vi "LINXx - Analog IO.vi"() -> ()   [LabVIEW 2019]
uses:
  <vilib>/MakerHub/LINX/Public/Peripherals/Analog/Analog Read 1 Chan.vi
  <vilib>/MakerHub/LINX/Public/Peripherals/Analog/Analog Read N Chans.vi
  <vilib>/MakerHub/LINX/Private/Local IO/LinxAnalogRead.vi
  <vilib>/MakerHub/LINX/Public/Utilities/Check Channel.vi
  <vilib>/MakerHub/LINX/Public/Utilities/Open Serial.vi
  <vilib>/MakerHub/LINX/Public/Peripherals/Analog/Analog Write 1 Chan.vi
  <vilib>/MakerHub/LINX/Private/Utilties/Generate Error.vi
  <vilib>/MakerHub/LINX/LMH-LINX.lvlib
  vi.lib/LINXx/LINXx.lvlib
panel:
  in  "AI Channel":u8=15
  in  "AO Channel":u8=14
  in  "iterations per cycle":i32=400
  out "Loop Rate (Hz)":u32
  out "Waveform Chart":cluster{dbl, "Voltage":dbl}(graph)
  in  "Serial Port":refnum<visa-resource-name>="N/A"
  in  "stop":bool
  # "Setup"
  # "Wiring: connect selected input and output \npins together"
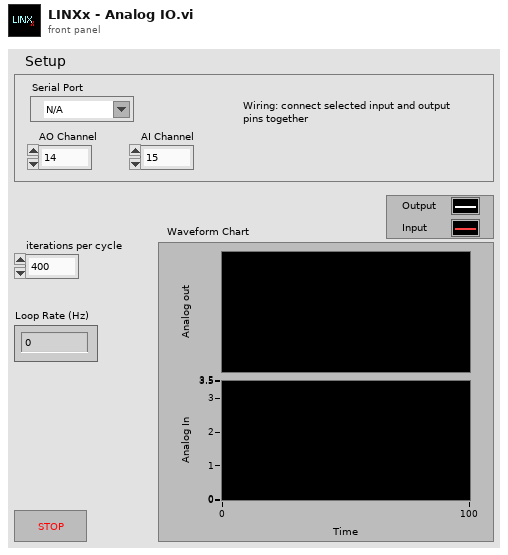
[diagram p1: front panel]
types:
  T1 = typedef "LMH-LINX.lvlib/LINX Ref.ctl" = cluster{"IO":T2, "Interface":T3, "LINX Device Config":T4}
  T2 = typedef "LMH-LINX.lvlib/Platform.ctl" = enum16{"Remote", "Local"}
  T3 = typedef "LMH-LINX.lvlib/Interface.ctl" = enum16{"Serial", "TCP"}
  T4 = typedef "LMH-LINX.lvlib/Device.lvlib/LINX Device Config.ctl" = cluster{"Interface":T3, "COM Port":refnum<visa-resource-name>, "TCP Configuration":T5, "Device Family":u8, "Device ID":u8, "Device Name":string, "TCP Ref":refnum<k5>, "Channels":T6}
  T5 = typedef "LMH-LINX.lvlib/Device.lvlib/TCP Config.ctl" = cluster{"IP Address":string, "Port":u16}
  T6 = typedef "LMH-LINX.lvlib/Channels.ctl" = cluster{"DI":u8[], "DO":u8[], "AI":u8[], "AO":u8[], "PWM":u8[], "QE":u8[], "UART":u8[], "I2C 2":u8[], "SPI":u8[], "CAN":u8[], "Servo":u8[], "AI Ref (V)":dbl, "AI Resolution (Bits)":u8, "AO Ref (V)":dbl, "AO Resolution (Bits)":u8}
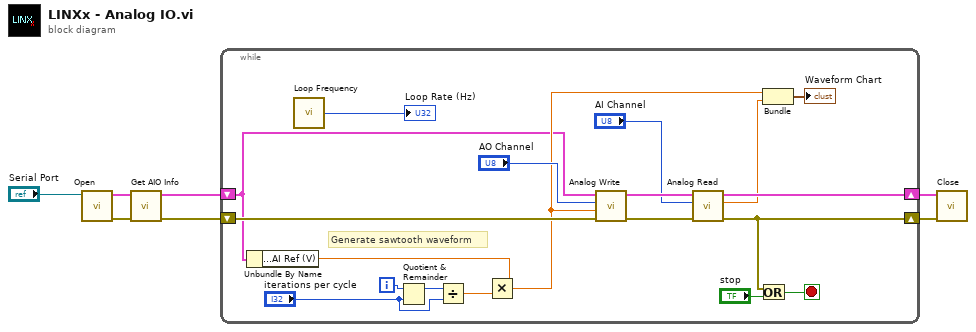
[diagram p0: block diagram]
diagram:
  n1 = call-poly <vilib>:"Open.vi"("Serial Port"="Serial Port") -> ("Error Out"=w4:errorcluster, "LINX Resource"=w3:T1)  [unwired: 8 in, 1 out]
  n2 = call "Get AIO Info.vi"("Error In"=w4, "LINX Resource"=w3) -> ("Error Out"=w1:errorcluster, "LINX resource"=w2:T1)  [unwired: 6 in, 2 out]
  n3 = while {
    shift-right: [w17] -> w7
    shift-left: w2 -> [w9]
    shift-right: [w21] -> w6
    shift-left: w1 -> [w26]
    i -> [w24]
    stop <- w22 stop-if-true
    # "Generate sawtooth waveform"
    n4 = Unbundle By Name(w9) -> ("LINX Device Config.Channels.AI Ref (V)"=w8:dbl)
    n5 = call <vilib>:"Loop Frequency.vi"() -> ("Loop Rate (Hz)"=→"Loop Rate (Hz)":u32)
    n6 = Quotient & Remainder(x=w24, y="iterations per cycle") -> (x-y*floor(x/y)=w13:i32)  [unwired: 1 out]
    n7 = Divide(x=w13, y="iterations per cycle") -> (x/y=w12:dbl)
    n8 = Multiply(x=w8, y=w12) -> (x*y=w11:dbl)
    n9 = call-poly <vilib>:"Analog Write.vi"("Error In"=w26, "AO Value"=w11, "AO Channel"="AO Channel", "LINX Resource"=w9) -> ("Error Out"=w20:errorcluster, "LINX Resource"=w19:T1)  [unwired: 6 in]
    n10 = call-poly <vilib>:"Analog Read.vi"("Error In"=w20, "Analog Channel"="AI Channel", "LINX Resource"=w19) -> ("Error Out"=w21:errorcluster, "Voltage"=w10:dbl, "LINX Resource"=w17:T1)  [unwired: 5 in, 1 out]
    n11 = Or(x=w21, y="stop") -> (x .or. y?=w22:bool)
    n12 = Bundle(w11, "Voltage"=w10) -> (→"Waveform Chart":cluster{dbl, "Voltage":dbl})  [unwired: 1 in]
  }
  n13 = call <vilib>:"Close.vi"("Error In"=w6, "LINX Resource"=w7) -> ()  [unwired: 9 in, 1 out]
